vi "Add Transfer.vi"(4 "inline":bool, 6 "Group Decimation (1)":u64, 8 "error in (no error)":errorcluster, 9 "Transfer":refnum<class "Transfer.lvclass">, 10 "parent tag":string, 11 "Application Data In":T1) -> (0 "error out":errorcluster, 3 "Application Data Out":T1)   [LabVIEW 2017, in "DSF Data Viewer.lvlib"]
uses:
  DSF Data Viewer.lvlib
  Main VI/Application Data.ctl
  Core/Engine/Classes/Framework/Framework.lvclass
  <vilib>/NI/Memory Manager/Classes/Pointer/Pointer.lvclass
  Buffer Reader/Buffer Data.ctl
  Core/Engine/Classes/Buffer/Buffer.lvclass
  Core/Engine/Classes/Transfer/Transfer.lvclass
  Core/Engine/Classes/Transfer/Transfer.lvclass/Transfer.ctl
  ID to Tree Items/Tree Item Type.ctl
  Core/Engine/Classes/Buffer/Buffers.lvclass/Buffers.ctl
  Core/Engine/Classes/Buffer/Get Async Buffer.vi
  Core/Engine/Classes/Buffer/Get String Buffer.vi
  Core/Engine/Classes/Buffer/Get Inline Buffer.vi
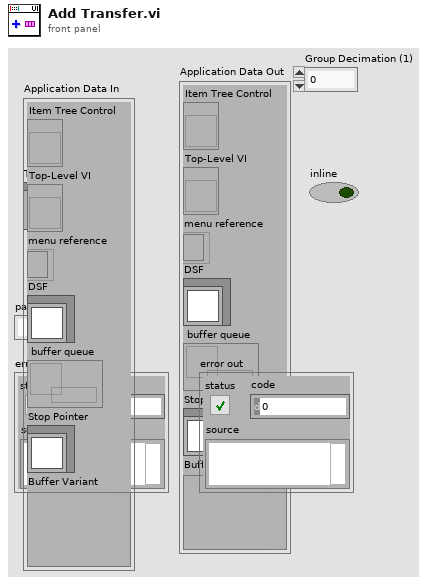
[diagram p1: front panel]
types:
  T1 = typedef "DSF Data Viewer.lvlib/Application Data.ctl" = cluster{"Item Tree Control":refnum<vi>, "Top-Level VI":refnum<vi>, "menu reference":refnum<k9>, "DSF":refnum<class "Framework.lvclass">, "buffer queue":refnum<queue>, "Stop Pointer":refnum<class "Pointer.lvclass">, "Buffer Variant":variant}
  T2 = typedef "DSF Data Viewer.lvlib/Buffer Data.ctl" = cluster{"Buffer":refnum<class "Buffer.lvclass">, "decimation":u64}
  T3 = typedef "DSF Data Viewer.lvlib/Tree Item Type.ctl" = enum16{"Framework", "Plugin Group", "Plugin", "Group", "Transfer", "Buffer", "Channel"}
  T4 = typedef "DSF Data Viewer.lvlib/Tree Item.ctl" = cluster{"Left Cell String":string, "Child Text":string[], "Child Tag":string, "Glyph Index":i32}
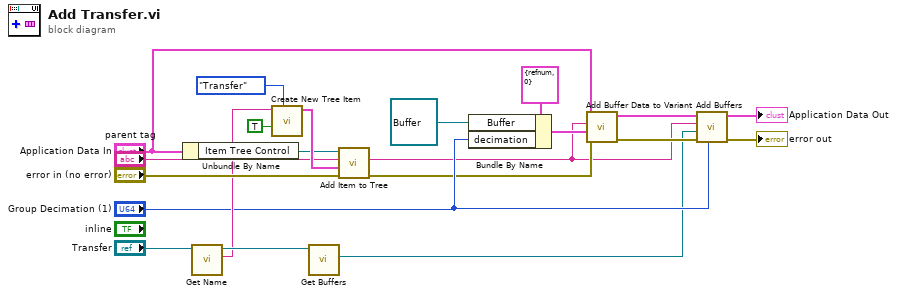
[diagram p0: block diagram]
diagram:
  n1 = Unbundle By Name("Application Data In") -> ("Item Tree Control"=w13:refnum<vi>)
  n2 = call "Get Name.vi"("Transfer in"="Transfer") -> ("name"=w14:string, "Transfer out"=w19:refnum<class "Transfer.lvclass">)  [unwired: 9 in]
  n3 = call "Create New Tree Item.vi"("Item Type"=Tree_Item_Type."Transfer", "found?"=TRUE, "Left Cell String"=w14) -> ("Item"=w21:T4)  [unwired: 7 in, 1 out]
  n4 = call "Get Buffers.vi"("Transfer in"=w19) -> ("Buffers"=w4:refnum<class "Buffers.lvclass">)  [unwired: 9 in, 1 out]
  n5 = call "Add Item to Tree.vi"("error in (no error)"="error in (no error)", "Item"=w21, "parent tag"="parent tag", "TreeControl in"=w13) -> ("error out"=w5:errorcluster, "new item tag"=w3:string)  [unwired: 5 in, 1 out]
  n6 = Bundle By Name(cluster=T2 {"Buffer"=refnum, "decimation"=0} ("Buffer data"), "Buffer"=refnum<class "Buffer.lvclass"> refnum, "decimation"="Group Decimation (1)") -> (w12:T2)
  n7 = call "Add Buffer Data to Variant.vi"("error in (no error)"=w5, "Buffer data"=w12, "tag"=w3, "Application Data In in"="Application Data In") -> ("error out"=w8:errorcluster, "Application Data In out"=w6:T1)  [unwired: 6 in]
  n8 = call "Add Buffers.vi"("Decimation"="Group Decimation (1)", "error in (no error)"=w8, "Buffers"=w4, "parent tag"=w3, "Application Data In"=w6) -> ("error out"=→"error out":errorcluster, "Application Data out"=→"Application Data Out":T1)  [unwired: 5 in]
